vi "1. Main demo.vi"() -> ()   [LabVIEW 2020]
uses:
  UnderAutomation.Yaskawa/UnderAutomation.Yaskawa.lvlib
  C:/Users/fg/Documents/Yaskawa.vi/LabVIEW_2024/UnderAutomation.Yaskawa/lib/UnderAutomation.Yaskawa.dll
  LabVIEW_2024/UnderAutomation.Yaskawa/lib/UnderAutomation.Yaskawa.dll
panel:
  out "HighSpeedEServer":refnum<k24>
  out "Connected":bool
  in  "Tab Control":T1(tab)
  in  "Disconnect":bool
  in  "Test":bool
  in  "Key":string
  in  "Licensee":string
  in  "Connect":bool
  in  "IP":string caption="Robot IP Address"
  out "License state":string
  out "Connect error":string
  out "Wwarning 1":string
  out "Name":string
  out "Parameter":string
  out "Software Version":string
  in  "Get status information":bool
  in  "Display":bool
  in  "Get Alarm":bool
  in  "Alarm Reset":bool
  in  "alarm":i32(ring)=1 items=["Latest"=1, "SecondLatest"=2, "ThirdLatest"=3, "FourthLatest"=4]
  out "Type":i32
  out "Text":string
  out "OccurringTime":string
  in  "Message":string
  out "Status":T2
  in  "Get System information":bool
  in  "Get executing job info":bool caption="Start job"
  in  "Servo off":bool
  in  "Servo on":bool
  in  "Start job":bool
  in  "Select job":bool caption="Start job"
  in  "Switching command":bool caption="Start job"
  in  "Job":string
  in  "Command":i32(ring)=1 items=["Cycle"=1, "Step"=2, "Continue"=3]
  in  "Line":i32
  out "Wwarning 2":string
  out "Name":string
  out "Line 2":i32
  out "SpeedOverride":i32
  out "Step":i32
  out "Wwarning 3":string
  out "Files":string[](array[string])
  in  "Pattern":string(combo)
  in  "Get file list":bool
  in  "Delete file":bool
  in  "Load file":bool
  in  "Get file":bool
  in  "Name":string
  in  "Content":string
  out "Wwarning 4":string
  in  "Get cartesian position":bool
  in  "Get torque":bool
  in  "Get joint position":bool
  in  "Move joints":bool
  in  "Move Cartesian":bool
  in  "Speed":cluster{"classification":i32, "speed":dbl} {"classification" items=["LinkPercent", "Cartesian_MM_S", "Cartesian_DEG_S"]}
  in  "Axes Pulse":i32[](array[numeric])
  in  "Coordinate":cluster{"userCoordinate":i32, "coordinate":i32}={"userCoordinate"=0, "coordinate"=16} {"coordinate" items=["Base"=16, "Robot"=17, "User"=18, "Tool"=19]}
  in  "tool":i32
  in  "RCONF":i32
  in  "Pose":T3
  out "Torque":i32[](array[numeric])
  out "Wwarning 5":string
  in  "firstIndex":i32
  in  "count":i32
  in  "Read IO":bool
  in  "Read registers":bool
  in  "count":i32
  in  "firstIndex":i32
  in  "Read position variables":bool
  in  "count":i32
  in  "firstIndex":i32
  out "Value":u8[](array[numeric])
  out "Axes":i32[][](array[numeric])
  out "Value":u16[](array[numeric])
  in  "stop":bool
  # "UnderAutomation"
  # "https://underautomation.com/yaskawa"
  # "+"
  # "LabVIEW demo app for remote control and monitoring of your Yaskawa robot"
  # "Connect to robot"
  # "2. Ensure you have a trial or lifetime valid license"
  # "1. Set Yaskawa robot address"
  # "This is a commercial library, you have a 30-day trial period. But you can use it forever if you buy a perpetual licence for your company (regardless of the number of robot, applications or developers)."
  # "If you have a license :"
  # "3. Connect to the robot"
  # "Robot alarms and status"
  # "Alarms"
  # "Display on pendant"
  # "Status information"
  # "System information"
  # "Servo and job commands"
  # "Servo command"
  # "Start job"
  # "Executing job"
  # "Switch command"
  # "File handling"
  # "List  files"
  # "Edit  files"
  # "Current position and move"
  # "Current Torque"
  # "Joints"
  # "Cartesian"
  # "Read and Write registers"
  # "IO"
  # "Registers"
  # "Positions"
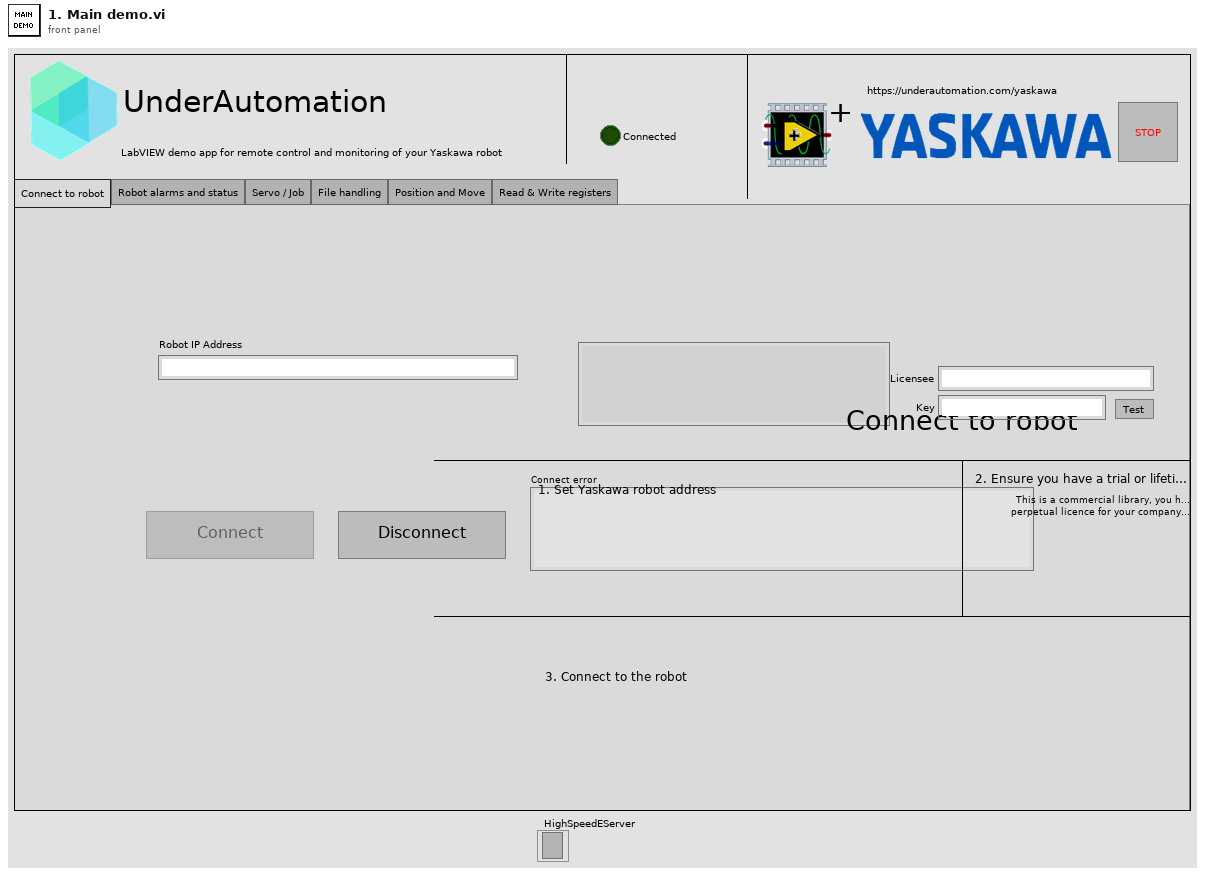
[diagram p1: front panel]
types:
  T1 = enum32{"Connect to robot", "Robot alarms and status", "Servo / Job", "File handling", "Position and Move", "Read & Write registers"}
  T2 = cluster{"Alarming":bool, "Automatic":bool, "CommandRemote":bool, "Cycle":bool, "ErrorOccurring":bool, "InGuardSafeOperation":bool, "InHoldStatusByCommand":bool, "InHoldStatusExternally":bool, "InHoldStatusPendant":bool, "Play":bool, "Running":bool, "ServoOn":bool, "Step":bool, "Teach":bool}
  T3 = cluster{"X":dbl, "Y":dbl, "Z":dbl, "Rx":dbl, "Ry":dbl, "Rz":dbl}
  T4 = enum8{"Enabled", "Disabled", "Disabled and Grayed Out"}
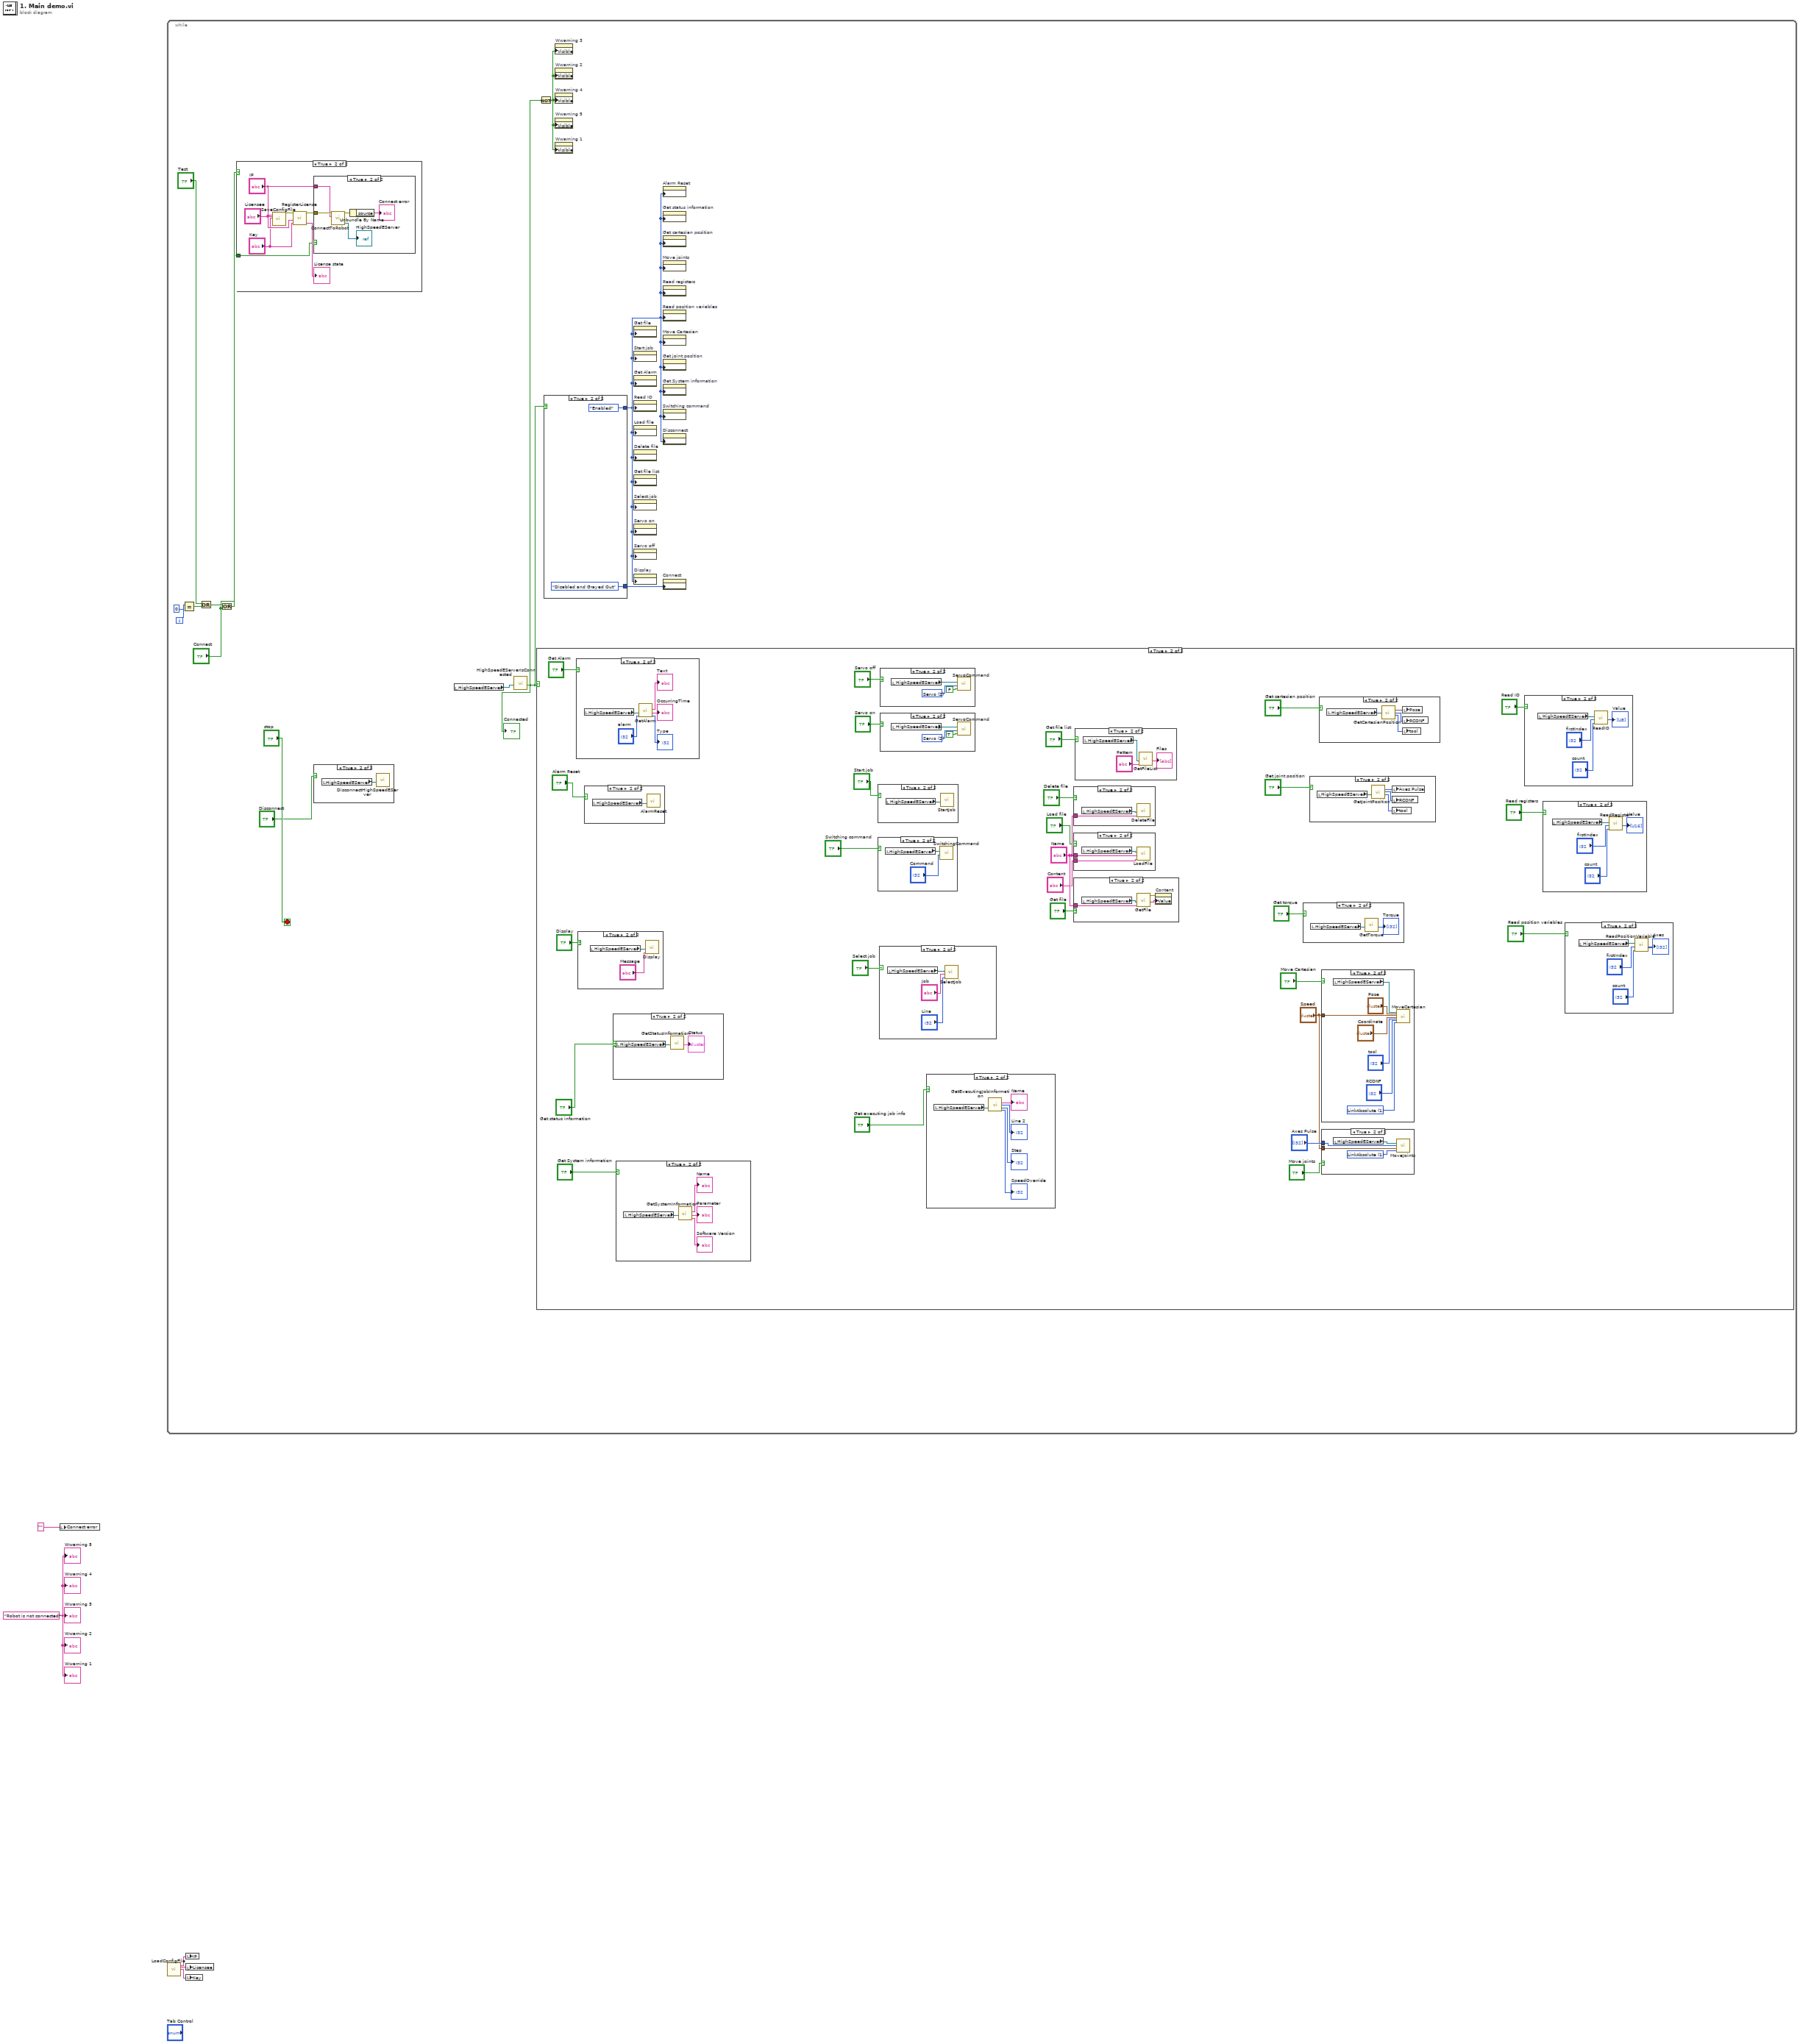
[diagram p0: block diagram]
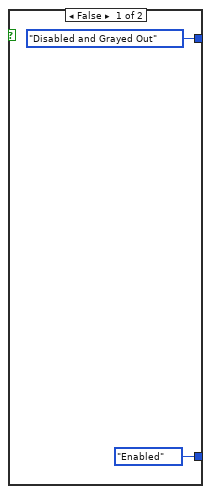
[diagram p3: hidden frame]
diagram:
  w2 = "Robot is not connected" ("Wwarning 1")
  n1 = local write "Connect error"("" ("Connect error")) -> ()
  n2 = while {
    i -> [w17]
    stop <- "stop" stop-if-true
    n3 = Equal?(x=w17, y=0) -> (x = y?=w15:bool)
    n4 = Or(x="Test", y=w15) -> (x .or. y?=w14:bool)
    n5 = Or(x=w14, y="Connect") -> (x .or. y?=w13:bool)
    n6 = case shown="True" w13 {
      tunnel: "Connect" -> [_ w128]
      frame False {
      }
      frame True {
        n7 = call "SaveConfigFile.vi"("IP"="IP", "Licensee"="Licensee", "Key"="Key") -> ("error out"=w131:errorcluster)  [unwired: 24 in]
        n8 = call "RegisterLicense.vi"("key"="Key", "Licensee"="Licensee", "error in (no error)"=w131) -> ("License state"=→"License state":string, "error out"=w130:errorcluster)  [unwired: 6 in, 1 out]
        n9 = case shown="True" w128 {
          tunnel: w130 -> [_ w139]
          tunnel: "IP" -> [_ w138]
          frame False {
          }
          frame True {
            n10 = call "ConnectToRobot.vi"("ip"=w138, "error in (no error)"=w139) -> ("HighSpeedEServer"=→"HighSpeedEServer":refnum<k24>, "error out"=w137:errorcluster)  [unwired: 7 in]
            n11 = Unbundle By Name(w137) -> ("source"=→"Connect error":string)
          }
        }
      }
    }
    n12 = case shown="True" "Disconnect" {
      frame False {
      }
      frame True {
        n13 = local read "HighSpeedEServer"() -> (w20:refnum<k24>)
        n14 = call "DisconnectHighSpeedEServer.vi"("HighSpeedEServer"=w20) -> ()  [unwired: 10 in, 1 out]
      }
    }
    n15 = local read "HighSpeedEServer"() -> (w11:refnum<k24>)
    n16 = call "HighSpeedEServerIsConnected.vi"("HighSpeedEServer"=w11) -> ("Connected"=w8:bool)  [unwired: 9 in, 1 out]
    "Connected" <- w8
    n17 = case shown="True" w8 {
      frame False {
      }
      frame True {
        n18 = case shown="True" "Get Alarm" {
          frame False {
          }
          frame True {
            n19 = local read "HighSpeedEServer"() -> (w127:refnum<k24>)
            n20 = call "GetAlarm.vi"("alarm"="alarm", "HighSpeedEServer"=w127) -> ("Type"=→"Type":i32, "OccurringTime"=→"OccurringTime":string, "Text"=→"Text":string)  [unwired: 6 in, 1 out]
          }
        }
        n21 = case shown="True" "Display" {
          frame False {
          }
          frame True {
            n22 = local read "HighSpeedEServer"() -> (w121:refnum<k24>)
            n23 = call "Display.vi"("message"="Message", "HighSpeedEServer"=w121) -> ()  [unwired: 9 in, 1 out]
          }
        }
        n24 = case shown="True" "Alarm Reset" {
          frame False {
          }
          frame True {
            n25 = local read "HighSpeedEServer"() -> (w122:refnum<k24>)
            n26 = call "AlarmReset.vi"("HighSpeedEServer"=w122) -> ()  [unwired: 10 in, 1 out]
          }
        }
        n27 = case shown="True" "Get status information" {
          frame False {
          }
          frame True {
            n28 = local read "HighSpeedEServer"() -> (w119:refnum<k24>)
            n29 = call "GetStatusInformation.vi"("HighSpeedEServer"=w119) -> ("Status"=→"Status":T2)  [unwired: 9 in, 1 out]
          }
        }
        n30 = case shown="True" "Get System information" {
          frame False {
          }
          frame True {
            n31 = local read "HighSpeedEServer"() -> (w117:refnum<k24>)
            n32 = call "GetSystemInformation.vi"("HighSpeedEServer"=w117) -> ("SoftwareVersion"=→"Software Version":string, "Parameter"=→"Parameter":string, "Name"=→"Name":string)  [unwired: 7 in, 1 out]
          }
        }
        n33 = case shown="True" "Switching command" {
          frame False {
          }
          frame True {
            n34 = local read "HighSpeedEServer"() -> (w106:refnum<k24>)
            n35 = call "SwitchingCommand.vi"("command"="Command", "HighSpeedEServer"=w106) -> ()  [unwired: 9 in, 1 out]
          }
        }
        n36 = case shown="True" "Start job" {
          frame False {
          }
          frame True {
            n37 = local read "HighSpeedEServer"() -> (w107:refnum<k24>)
            n38 = call "StartJob.vi"("HighSpeedEServer"=w107) -> ()  [unwired: 10 in, 1 out]
          }
        }
        n39 = case shown="True" "Select job" {
          frame False {
          }
          frame True {
            n40 = local read "HighSpeedEServer"() -> (w104:refnum<k24>)
            n41 = call "SelectJob.vi"("line"="Line", "job"="Job", "HighSpeedEServer"=w104) -> ()  [unwired: 8 in, 1 out]
          }
        }
        n42 = case shown="True" "Servo off" {
          frame False {
          }
          frame True {
            w109 = u8 2 items=["Hold"=1, "Servo"=2, "HLock"=3] ("command")
            n43 = local read "HighSpeedEServer"() -> (w108:refnum<k24>)
            n44 = call "ServoCommand.vi"("value"=FALSE, "command"=w109, "HighSpeedEServer"=w108) -> ()  [unwired: 8 in, 1 out]
          }
        }
        n45 = case shown="True" "Servo on" {
          frame False {
          }
          frame True {
            w112 = u8 2 items=["Hold"=1, "Servo"=2, "HLock"=3] ("command")
            n46 = local read "HighSpeedEServer"() -> (w111:refnum<k24>)
            n47 = call "ServoCommand.vi"("value"=TRUE, "command"=w112, "HighSpeedEServer"=w111) -> ()  [unwired: 8 in, 1 out]
          }
        }
        n48 = case shown="True" "Get executing job info" {
          frame False {
          }
          frame True {
            n49 = local read "HighSpeedEServer"() -> (w56:refnum<k24>)
            n50 = call "GetExecutingJobInformation.vi"("HighSpeedEServer"=w56) -> ("Name"=→"Name":string, "Line"=→"Line 2":i32, "Step"=→"Step":i32, "SpeedOverride"=→"SpeedOverride":i32)  [unwired: 10 in, 1 out]
          }
        }
        n51 = case shown="True" "Delete file" {
          tunnel: "Name" -> [_ w98]
          frame False {
          }
          frame True {
            n52 = local read "HighSpeedEServer"() -> (w97:refnum<k24>)
            n53 = call "DeleteFile.vi"("name"=w98, "HighSpeedEServer"=w97) -> ()  [unwired: 9 in, 1 out]
          }
        }
        n54 = case shown="True" "Load file" {
          tunnel: "Name" -> [_ w92]
          tunnel: "Content" -> [_ w91]
          frame False {
          }
          frame True {
            n55 = local read "HighSpeedEServer"() -> (w90:refnum<k24>)
            n56 = call "LoadFile.vi"("content"=w91, "name"=w92, "HighSpeedEServer"=w90) -> ()  [unwired: 8 in, 1 out]
          }
        }
        n57 = case shown="True" "Get file" {
          tunnel: "Name" -> [_ w96]
          frame False {
          }
          frame True {
            n58 = local read "HighSpeedEServer"() -> (w93:refnum<k24>)
            n59 = call "GetFile.vi"("name"=w96, "HighSpeedEServer"=w93) -> ("Content"=w95:string, "error out"=w94:errorcluster)  [unwired: 8 in]
            n60 = property on="Content" class="Str"(error in=w94, "Value"=w95) -> ()  [unwired: 1 in, 2 out]
          }
        }
        n61 = case shown="True" "Get file list" {
          frame False {
          }
          frame True {
            n62 = local read "HighSpeedEServer"() -> (w100:refnum<k24>)
            n63 = call "GetFileList.vi"("pattern"="Pattern", "HighSpeedEServer"=w100) -> ("Files"=→"Files":string[])  [unwired: 8 in, 1 out]
          }
        }
        n64 = case shown="True" "Get torque" {
          frame False {
          }
          frame True {
            n65 = local read "HighSpeedEServer"() -> (w81:refnum<k24>)
            n66 = call "GetTorque.vi"("HighSpeedEServer"=w81) -> ("Axes"=→"Torque":i32[])  [unwired: 9 in, 1 out]
          }
        }
        n67 = case shown="True" "Get joint position" {
          frame False {
          }
          frame True {
            n68 = local read "HighSpeedEServer"() -> (w85:refnum<k24>)
            n69 = call "GetJointPosition.vi"("HighSpeedEServer"=w85) -> ("Axes"=w84:i32[], "RCONF"=w83:i32, "ToolNumber"=w82:i32)  [unwired: 10 in, 2 out]
            n70 = local write "Axes Pulse"(w84) -> ()
            n71 = local write "RCONF"(w83) -> ()
            n72 = local write "tool"(w82) -> ()
          }
        }
        n73 = case shown="True" "Get cartesian position" {
          frame False {
          }
          frame True {
            n74 = local read "HighSpeedEServer"() -> (w89:refnum<k24>)
            n75 = call "GetCartesianPosition.vi"("HighSpeedEServer"=w89) -> ("Pose"=w88:T3, "RCONF"=w87:i32, "ToolNumber"=w86:i32)  [unwired: 10 in, 2 out]
            n76 = local write "Pose"(w88) -> ()
            n77 = local write "RCONF"(w87) -> ()
            n78 = local write "tool"(w86) -> ()
          }
        }
        n79 = case shown="True" "Move Cartesian" {
          tunnel: "Speed" -> [_ w78]
          frame False {
          }
          frame True {
            w74 = 1 items=["LinkAbsolute"=1, "StraightAbsolute"=2, "StraightIncrement"=3] ("commandtype")
            n80 = local read "HighSpeedEServer"() -> (w79:refnum<k24>)
            n81 = call "MoveCartesian.vi"("HighSpeedEServer"=w79, "Pose"="Pose", "Speed"=w78, "Coordinate"="Coordinate", "tool"="tool", "RCONF"="RCONF", "commandtype"=w74) -> ()  [unwired: 20 in, 1 out]
          }
        }
        n82 = case shown="True" "Move joints" {
          tunnel: "Axes Pulse" -> [_ w71]
          tunnel: "Speed" -> [_ w69]
          frame False {
          }
          frame True {
            w70 = 1 items=["LinkAbsolute"=1, "StraightAbsolute"=2, "StraightIncrement"=3] ("commandtype")
            n83 = local read "HighSpeedEServer"() -> (w72:refnum<k24>)
            n84 = call "MoveJoints.vi"("HighSpeedEServer"=w72, "axesPulse"=w71, "Speed"=w69, "commandtype"=w70) -> ()  [unwired: 11 in, 1 out]
          }
        }
        n85 = case shown="True" "Read IO" {
          frame False {
          }
          frame True {
            n86 = local read "HighSpeedEServer"() -> (w68:refnum<k24>)
            n87 = call "ReadIO.vi"("count"="count", "firstIndex"="firstIndex", "HighSpeedEServer"=w68) -> ("Value"=→"Value":u8[])  [unwired: 7 in, 1 out]
          }
        }
        n88 = case shown="True" "Read registers" {
          frame False {
          }
          frame True {
            n89 = local read "HighSpeedEServer"() -> (w64:refnum<k24>)
            n90 = call "ReadRegister.vi"("count"="count", "firstIndex"="firstIndex", "HighSpeedEServer"=w64) -> ("Value"=→"Value":u16[])  [unwired: 7 in, 1 out]
          }
        }
        n91 = case shown="True" "Read position variables" {
          frame False {
          }
          frame True {
            n92 = local read "HighSpeedEServer"() -> (w60:refnum<k24>)
            n93 = call "ReadPositionVariable.vi"("count"="count", "firstIndex"="firstIndex", "HighSpeedEServer"=w60) -> ("Axes"=→"Axes":i32[][])  [unwired: 7 in, 1 out]
          }
        }
      }
    }
    n94 = Not(x=w8) -> (.not. x?=w7:bool)
    n95 = case shown="True" w8 {
      tunnel: [T4."Enabled" ("Disabled") T4."Disabled and Grayed Out" ("Disabled")] -> w10
      tunnel: [T4."Disabled and Grayed Out" ("Disabled") T4."Enabled" ("Disabled")] -> w6
      frame False {
      }
      frame True {
      }
    }
    n96 = property on="Wwarning 3" class="Str"("Visible"=w7) -> ()  [unwired: 2 in, 2 out]
    n97 = property on="Wwarning 2" class="Str"("Visible"=w7) -> ()  [unwired: 2 in, 2 out]
    n98 = property on="Wwarning 4" class="Str"("Visible"=w7) -> ()  [unwired: 2 in, 2 out]
    n99 = property on="Wwarning 5" class="Str"("Visible"=w7) -> ()  [unwired: 2 in, 2 out]
    n100 = property on="Wwarning 1" class="Str"("Visible"=w7) -> ()  [unwired: 2 in, 2 out]
    n101 = property on="Get file" class="Bool"("DisabledEnum"=w6) -> ()  [unwired: 2 in, 2 out]
    n102 = property on="Start job" class="Bool"("DisabledEnum"=w6) -> ()  [unwired: 2 in, 2 out]
    n103 = property on="Get Alarm" class="Bool"("DisabledEnum"=w6) -> ()  [unwired: 2 in, 2 out]
    n104 = property on="Read IO" class="Bool"("DisabledEnum"=w6) -> ()  [unwired: 2 in, 2 out]
    n105 = property on="Load file" class="Bool"("DisabledEnum"=w6) -> ()  [unwired: 2 in, 2 out]
    n106 = property on="Delete file" class="Bool"("DisabledEnum"=w6) -> ()  [unwired: 2 in, 2 out]
    n107 = property on="Get file list" class="Bool"("DisabledEnum"=w6) -> ()  [unwired: 2 in, 2 out]
    n108 = property on="Select job" class="Bool"("DisabledEnum"=w6) -> ()  [unwired: 2 in, 2 out]
    n109 = property on="Servo on" class="Bool"("DisabledEnum"=w6) -> ()  [unwired: 2 in, 2 out]
    n110 = property on="Servo off" class="Bool"("DisabledEnum"=w6) -> ()  [unwired: 2 in, 2 out]
    n111 = property on="Display" class="Bool"("DisabledEnum"=w6) -> ()  [unwired: 2 in, 2 out]
    n112 = property on="Alarm Reset" class="Bool"("DisabledEnum"=w6) -> ()  [unwired: 2 in, 2 out]
    n113 = property on="Get status information" class="Bool"("DisabledEnum"=w6) -> ()  [unwired: 2 in, 2 out]
    n114 = property on="Get cartesian position" class="Bool"("DisabledEnum"=w6) -> ()  [unwired: 2 in, 2 out]
    n115 = property on="Move joints" class="Bool"("DisabledEnum"=w6) -> ()  [unwired: 2 in, 2 out]
    n116 = property on="Read registers" class="Bool"("DisabledEnum"=w6) -> ()  [unwired: 2 in, 2 out]
    n117 = property on="Read position variables" class="Bool"("DisabledEnum"=w6) -> ()  [unwired: 2 in, 2 out]
    n118 = property on="Move Cartesian" class="Bool"("DisabledEnum"=w6) -> ()  [unwired: 2 in, 2 out]
    n119 = property on="Get joint position" class="Bool"("DisabledEnum"=w6) -> ()  [unwired: 2 in, 2 out]
    n120 = property on="Get System information" class="Bool"("DisabledEnum"=w6) -> ()  [unwired: 2 in, 2 out]
    n121 = property on="Switching command" class="Bool"("DisabledEnum"=w6) -> ()  [unwired: 2 in, 2 out]
    n122 = property on="Disconnect" class="Bool"("DisabledEnum"=w6) -> ()  [unwired: 2 in, 2 out]
    n123 = property on="Connect" class="Bool"("DisabledEnum"=w10) -> ()  [unwired: 2 in, 2 out]
  }
  n124 = call "LoadConfigFile.vi"() -> ("IP"=w5:string, "Licensee"=w4:string, "Key"=w3:string)  [unwired: 24 in, 1 out]
  n125 = local write "IP"(w5) -> ()
  n126 = local write "Licensee"(w4) -> ()
  n127 = local write "Key"(w3) -> ()
  "Wwarning 1" <- w2
  "Wwarning 2" <- w2
  "Wwarning 3" <- w2
  "Wwarning 4" <- w2
  "Wwarning 5" <- w2
